vi "Channel 1 Image Ring.vi"() -> ()   [LabVIEW 2016]
uses:
  <vilib>/vision/Image Controls.llb/IMAQ Image.ctl
panel:
  in  "En Face Image":T1
  in  "Channel 1 Ring Size":dbl
  in  "Channel 1 Index":dbl
  in  "Channel 1 Image":T1[](array[typedef])
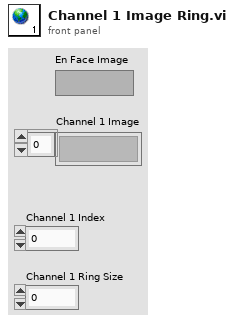
[diagram p1: front panel]
types:
  T1 = typedef "IMAQ Image.ctl" = refnum<image>
diagram:
